vi "kalman filter2.vi"(6 "Boolean":bool, 7 "iteração":dbl, 11 "z_k":T1) -> (3 "x_k|k":T1)   [LabVIEW 2016]
uses:
  <vilib>/Analysis/Matrix/Datatypes/RealMatrix.ctl
  <vilib>/Analysis/baseanly.llb/Real Inverse Matrix.vi
  <vilib>/Analysis/Matrix/Numeric/Multiply/Multiply - RM,RM.vi
  <vilib>/Analysis/Matrix/Numeric/Add/Add - RM,RM.vi
  <vilib>/Analysis/Matrix/NI_Matrix.lvlib
  <vilib>/Analysis/NI_AALBase.lvlib
panel:
  in  "Pk-1|k-1":T1
  out "Pk|k":T1
  out "K_k":T1
  out "Inverse Matrix":T1
  in  "x_k-1|k-1":T1
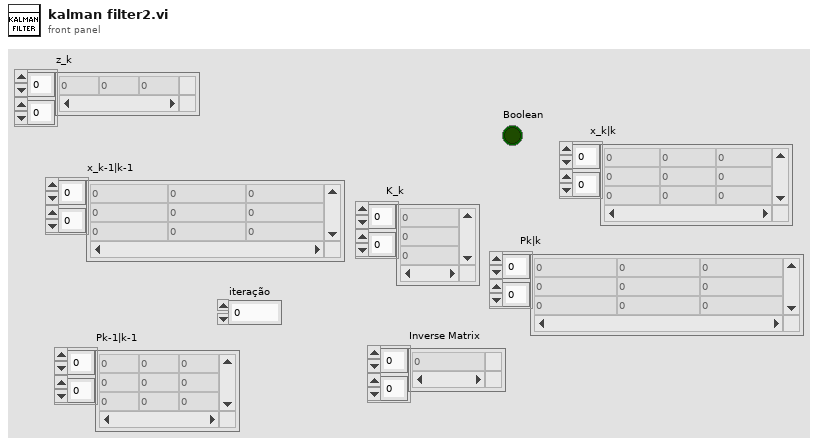
[diagram p1: front panel]
types:
  T1 = typedef "NI_Matrix.lvlib/RealMatrix.ctl" = dbl[][]
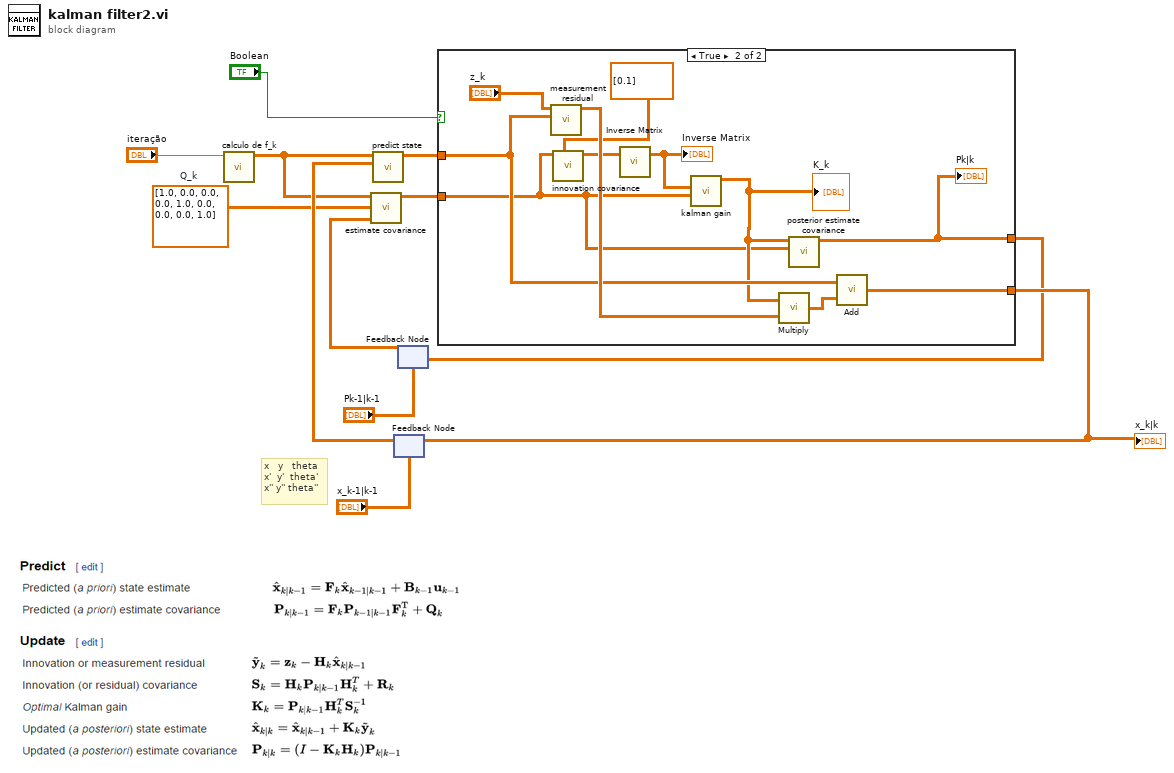
[diagram p0: block diagram]
diagram:
  w1 = T1 [[1.0, 0.0, 0.0], [0.0, 1.0, 0.0], [0.0, 0.0, 1.0]]  # Q_k
  # "x   y   theta\nx'  y'  theta'\nx'' y'' theta''"
  n1 = call "calculo de f_k.vi"("iteração"="iteração") -> ("F_k"=w6:T1)  [unwired: 10 in]
  n2 = feedback #1("x_k-1|k-1") -> (w8:T1)
  n3 = call "predict state.vi"("x_k-1|k-1"=w8, "F_k"=w6) -> ("x_k|k-1"=w7:T1)  [unwired: 9 in]
  n4 = feedback #2("Pk-1|k-1") -> (w5:T1)
  n5 = call "estimate covariance.vi"("Q_k"=w1, "Pk-1|k-1"=w5, "F_k"=w6) -> ("Pk|k-1"=w3:T1)  [unwired: 8 in]
  n6 = case shown="True" "Boolean" {
    tunnel: [w14 w24] -> w10
    tunnel: w7 -> [w14 w21]
    tunnel: [w13 w18] -> w4
    tunnel: w3 -> [w13 w16]
    frame False {
    }
    frame True {
      n7 = call "measurement residual.vi"("x_k|k-1"=w21, "z_k"="z_k") -> ("y~_k"=w23:T1)  [unwired: 9 in]
      n8 = call "innovation covariance.vi"("R"=T1 [[0.1]], "Pk|k-1"=w16) -> ("S_k"=w20:T1)  [unwired: 8 in, 1 out]
      n9 = call-poly <vilib>:"Inverse Matrix.vi"("Input Matrix"=w20) -> ("Inverse Matrix"=w19:T1)  [unwired: 1 in, 1 out]
      "Inverse Matrix" <- w19
      n10 = call "kalman gain.vi"("Pk|k-1"=w16, "S^-1"=w19) -> ("K_k"=w17:T1)  [unwired: 9 in]
      "K_k" <- w17
      n11 = call-poly <vilib>:"Multiply.vi"("Real Matrix B"=w23, "Real Matrix A"=w17) -> ("A * B"=w25:T1)
      n12 = call "posterior estimate covariance.vi"("Pk|k-1"=w16, "K_k"=w17) -> ("Pk|k"=w18:T1)  [unwired: 9 in]
      "Pk|k" <- w18
      n13 = call-poly <vilib>:"Add.vi"("Real Matrix B"=w25, "Real Matrix A"=w21) -> ("A + B"=w24:T1)
    }
  }
  "x_k|k" <- w10
  n14 = feedback-in #1(w10) -> ()
  n15 = feedback-in #2(w4) -> ()
